vi "Get Hash Info.vi"(8 "error in (no error)":errorcluster, 11 "MD5 in":refnum<class "MD5.lvclass">) -> (0 "error out":errorcluster, 1 "Output Length (Bytes)":i32, 2 "Blocksize (Bytes)":i32, 3 "MD5 out":refnum<class "MD5.lvclass">)   [LabVIEW 2017, in "Crypto.lvlib" / "MD5.lvclass"]
uses:
  MD5.lvclass
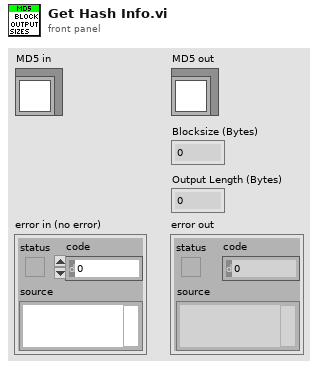
[diagram p1: front panel]
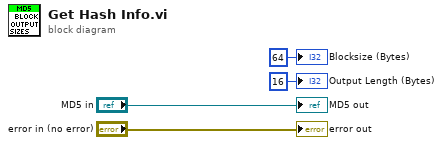
[diagram p0: block diagram]
diagram:
  "error out" <- "error in (no error)"
  "MD5 out" <- "MD5 in"
  "Blocksize (Bytes)" <- 64 ("Blocksize (Bytes)")
  "Output Length (Bytes)" <- 16 ("Output Length (Bytes)")
